vi "Simple Single Async.vi"(10 "B":dbl, 11 "A":dbl) -> (0 "error out":errorcluster, 3 "Future":refnum<class "Future.lvclass">)   [LabVIEW 2020, in "Futures-Examples.lvlib"]
uses:
  Futures-Examples.lvlib
  Promises/Promise/Promise.lvclass
  DoubleValue/DoubleValue.lvclass
  Simple Single Task.vi
  Promises/Future/Future.lvclass
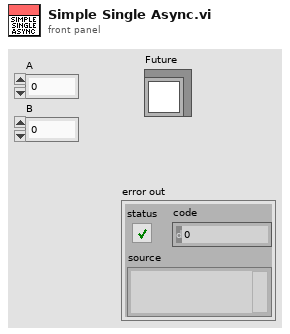
[diagram p1: front panel]
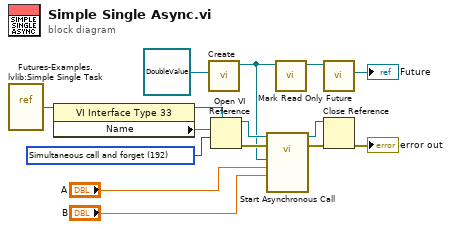
[diagram p0: block diagram]
diagram:
  w9 = 192 items=["Record modifications"=1, "Open templates for editing"=2, "Prompt user to save"=4, "Prepare for reentrant run"=8, "Prompt to find missing subVIs"=16, "Hide loading dialog box"=32, "Enable simultaneous calls"=64, "Prepare to call and forget"=128, "Simultaneous call and forget"=192, "Prepare to call and collect"=256, "Simultaneous call and collect"=320]
  n1 = vi-ref "Futures-Examples.lvlib:Simple Single Task.vi"() -> (w7:refnum<vi>)
  n2 = property class="VI Interface Type 33"(reference=w7) -> (reference out=w10:refnum<vi>, "Name"=w8:string)  [unwired: 1 in, 1 out]
  n3 = call "Create.vi"("Result Type"=refnum<class "DoubleValue.lvclass"> refnum ("Futures-Examples.lvlib:DoubleValue.lvclass")) -> ("Promise"=w6:refnum<class "Promise.lvclass">)  [unwired: 9 in, 1 out]
  n4 = Open VI Reference(type specifier VI Refnum (for type only)=w10, vi path=w8, options=w9) -> (vi reference=w12:refnum<vi>, error out=w11:errorcluster)  [unwired: 3 in]
  n5 = call-by-ref "Start Asynchronous Call"(reference=w12, error in=w11, "B"="B", "A"="A", "Promise"=w6) -> (reference out=w14:refnum<vi>, error out=w13:errorcluster)  [unwired: 9 in]
  n6 = call "Mark Read Only.vi"("Promise in"=w6) -> ("Promise out"=w2:refnum<class "Promise.lvclass">)  [unwired: 9 in, 1 out]
  n7 = call "Future.vi"("Promise in"=w2) -> ("Future"=→"Future":refnum<class "Future.lvclass">)  [unwired: 9 in, 1 out]
  n8 = Close Reference(reference=w14, error in (no error)=w13) -> (error out=→"error out":errorcluster)
